vi "AndorTest.vi"() -> ()   [LabVIEW 2014]
uses:
  <userlib>/atmcd64d.llb/AcquisitionMode_mode typedef.ctl
  <userlib>/atmcd64d.llb/ReadMode_mode typedef.ctl
  <userlib>/atmcd64d.llb/Shutter_mode typedef.ctl
  <userlib>/atmcd64d.llb/Shutter_type typedef.ctl
  <userlib>/atmcd64d.llb/TriggerMode_mode typedef.ctl
  <userlib>/atmcd64d.llb/Error Code Enum typedef.ctl
panel:
  out "Waveform Chart":i32[][](graph)
  out "SetStatus":bool
  out "SetOut":T1
  out "Timing":T2 {"kinetic" format="%.2f"; "accumulate" format="%.2f"; "exposure" format="%.2f"}
  in  "MultiTrack":cluster{"StartRow":i32, "EndRow":i32}={"StartRow"=1, "EndRow"=256}
  in  "AcqSet":T3={"openingtime"=20, "closingtime"=20, "ExposureTime"=0.01, "AccumCycTime"=0.0, "AccumCycNum"=1, "KineticNum"=1, "KineticTime"=0.0} {"KineticTime" format="%.2f"; "AccumCycTime" format="%.2f"; "ExposureTime" format="%.2f"}
  in  "Mode":T9={"AcqMode"=enum."Single Scan", "ReadMode"=enum."Image", "ShutterMode"=enum."Auto", "GateMode"=enum."TTL High", "TriggerMode"=enum."Internal"}
  out "error out":errorcluster
  out "ShutDown":cluster{"CoolOff":bool, "ShutDown":bool}
  in  "stop":bool
  out "CoolerON":T10
  out "CurrentTemp":i32
  in  "TargetTemp":i32
  out "Speeds":T11
  out "SoftWVersion":T12
  out "HardWVersion":T13
  out "DevSize":cluster{"xpixels":i32, "ypixels":i32}
  out "DevInit":bool
  out "GetStatus":T14
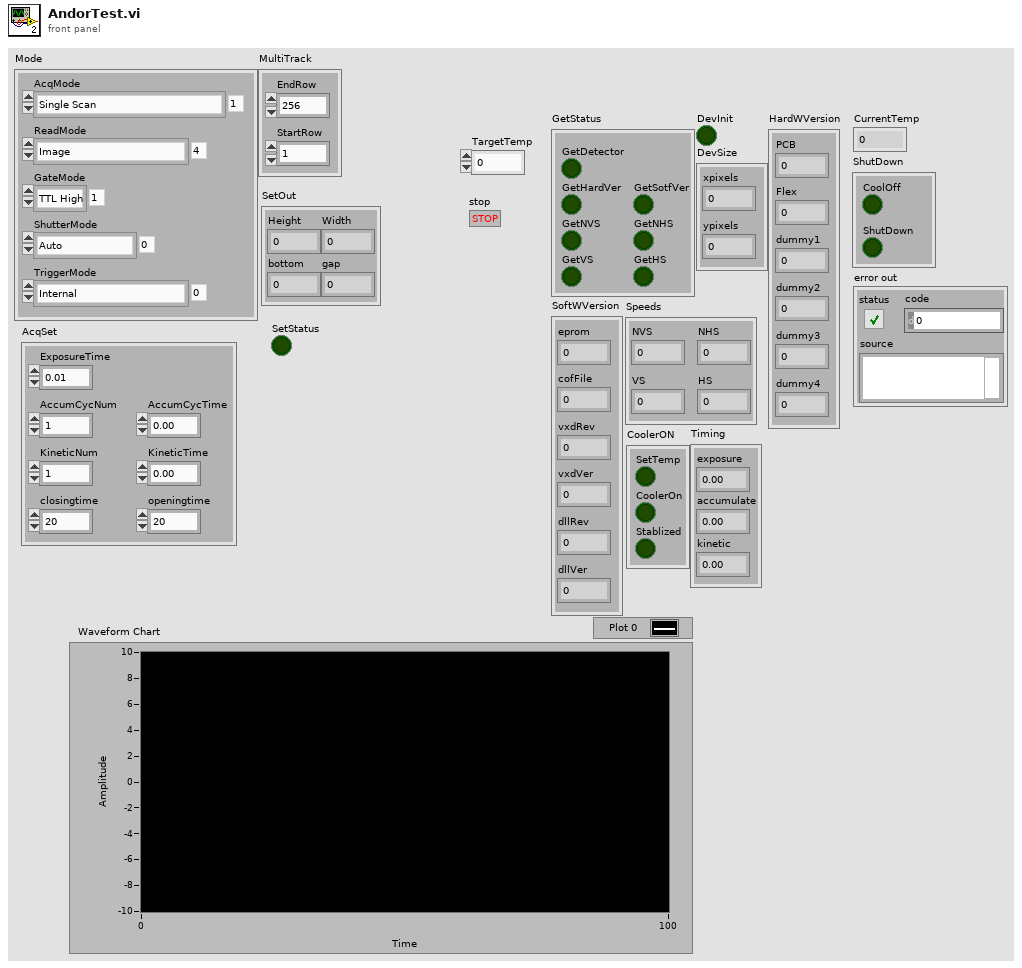
[diagram p1: front panel]
types:
  T1 = cluster{"Height":i32, "Width":i32, "bottom":i32, "gap":i32}
  T2 = cluster{"exposure":sgl, "accumulate":sgl, "kinetic":sgl}
  T3 = cluster{"openingtime":i32, "closingtime":i32, "ExposureTime":sgl, "AccumCycTime":sgl, "AccumCycNum":i32, "KineticNum":i32, "KineticTime":sgl}
  T4 = typedef "AcquisitionMode_mode typedef.ctl" = enum16{"Reserved (0)", "Single Scan", "Accumulate", "Kinetics", "Fast Kinetics", "Run Till Abort", "Reserved (6)", "Reserved (7)", "Reserved (8)", "Time Delayed Integration"}
  T5 = typedef "ReadMode_mode typedef.ctl" = enum16{"Full Vertical Binning", "Multi-Track", "Random-Track", "Single-Track", "Image"}
  T6 = typedef "Shutter_mode typedef.ctl" = enum16{"Auto", "Open", "Close", "N/A (3)", "Open FVB Series", "Open Any Series"}
  T7 = typedef "Shutter_type typedef.ctl" = enum16{"TTL Low", "TTL High"}
  T8 = typedef "TriggerMode_mode typedef.ctl" = enum16{"Internal", "External", "N/A (2)", "N/A (3)", "N/A (4)", "N/A (5)", "External Start", "External Exposure (Bulb)", "N/A (8)", "External FVB EM", "Software", "N/A (11)", "External Charge Shifting"}
  T9 = cluster{"AcqMode":T4, "ReadMode":T5, "ShutterMode":T6, "GateMode":T7, "TriggerMode":T8}
  T10 = cluster{"SetTemp":bool, "CoolerOn":bool, "Stablized":bool}
  T11 = cluster{"NVS":i32, "VS":i32, "NHS":dbl, "HS":i32}
  T12 = cluster{"eprom":u32, "cofFile":u32, "vxdRev":u32, "vxdVer":u32, "dllRev":u32, "dllVer":u32}
  T13 = cluster{"PCB":u32, "Flex":u32, "dummy1":u32, "dummy2":u32, "dummy3":u32, "dummy4":u32}
  T14 = cluster{"GetDetector":bool, "GetHardVer":bool, "GetNVS":bool, "GetVS":bool, "GetSotfVer":bool, "GetNHS":bool, "GetHS":bool}
  T15 = typedef "Error Code Enum typedef.ctl" = enum32{"N/A (0)", "DRV_ERROR_CODES", "DRV_SUCCESS", "DRV_VXDNOTINSTALLED", "DRV_ERROR_SCAN", "DRV_ERROR_CHECK_SUM", "DRV_ERROR_FILELOAD", "DRV_UNKNOWN_FUNC", "DRV_ERROR_VXD_INIT", "DRV_ERROR_ADDRESS", "DRV_ERROR_PAGELOCK", "DRV_ERROR_PAGEUNLOCK", "DRV_ERROR_BOARDTEST", "DRV_ERROR_ACK", "DRV_ERROR_UP_FIFO", "DRV_ERROR_PATTERN", "N/A (16)", "DRV_ACQUISITION_ERRORS", "DRV_ACQ_BUFFER", "DRV_ACQ_DOWNFIFO_FULL", "DRV_PROC_UNKONWN_INSTRUCTION", "DRV_ILLEGAL_OP_CODE", "DRV_KINETIC_TIME_NOT_MET", "DRV_ACCUM_TIME_NOT_MET", "DRV_NO_NEW_DATA", "N/A (25)", "DRV_SPOOLERROR", "N/A (27)", "N/A (28)", "N/A (29)", "N/A (30)", "N/A (31)", "N/A (32)", "DRV_TEMPERATURE_CODES", "DRV_TEMPERATURE_OFF", "DRV_TEMPERATURE_NOT_STABILIZED", "DRV_TEMPERATURE_STABILIZED", "DRV_TEMPERATURE_NOT_REACHED", "DRV_TEMPERATURE_OUT_RANGE", "DRV_TEMPERATURE_NOT_SUPPORTED", "DRV_TEMPERATURE_DRIFT", "N/A (41)", "N/A (42)", "N/A (43)", "N/A (44)", "N/A (45)", "N/A (46)", "N/A (47)", "N/A (48)", "DRV_GENERAL_ERRORS", "DRV_INVALID_AUX", "DRV_COF_NOTLOADED", "DRV_FPGAPROG", "DRV_FLEXERROR", "DRV_GPIBERROR", "N/A (55)", "N/A (56)", "N/A (57)", "N/A (58)", "N/A (59)", "N/A (60)", "N/A (61)", "N/A (62)", "N/A (63)", "DRV_DATATYPE", "DRV_DRIVER_ERRORS", "DRV_P1INVALID", "DRV_P2INVALID", "DRV_P3INVALID", "DRV_P4INVALID", "DRV_INIERROR", "DRV_COFERROR", "DRV_ACQUIRING", "DRV_IDLE", "DRV_TEMPCYCLE", "DRV_NOT_INITIALIZED", "DRV_P5INVALID", "DRV_P6INVALID", "DRV_INVALID_MODE", "DRV_INVALID_FILTER", "DRV_I2CERRORS", "DRV_I2CDEVNOTFOUND", "DRV_I2CTIMEOUT", "DRV_P7INVALID", "N/A (84)", "N/A (85)", "N/A (86)", "N/A (87)", "N/A (88)", "N/A (89)", "DRV_IOCERROR", "DRV_VRMVERSIONERROR"}
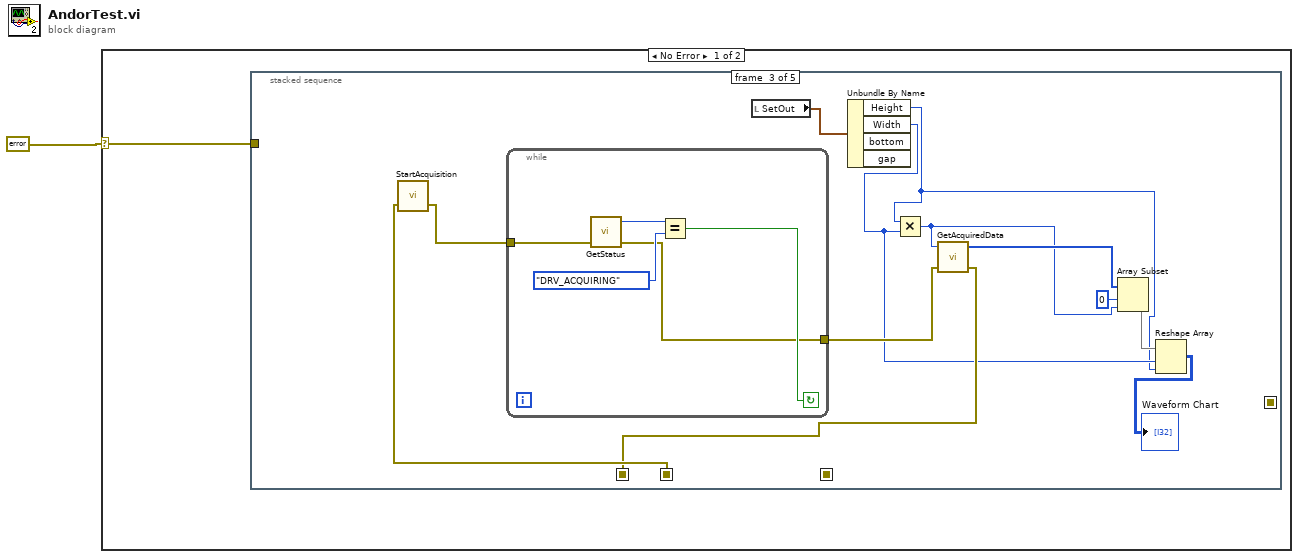
[diagram p0: block diagram]
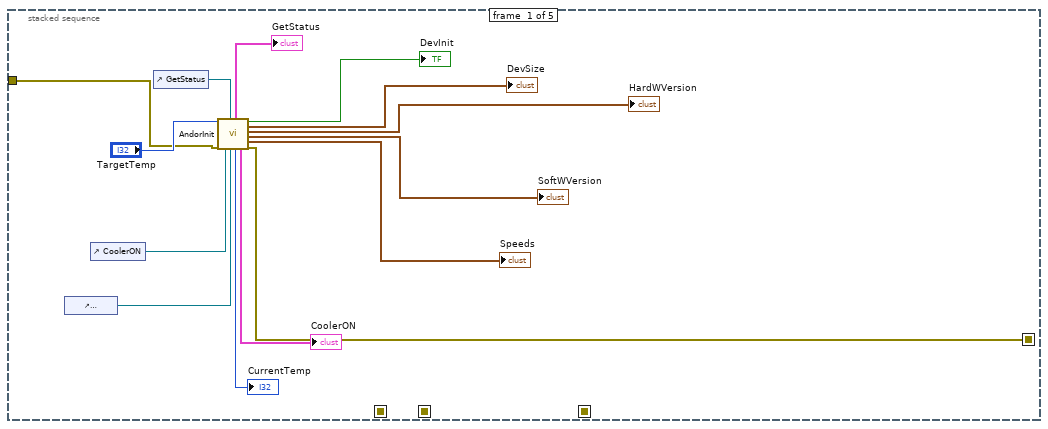
[diagram p2: hidden frame]
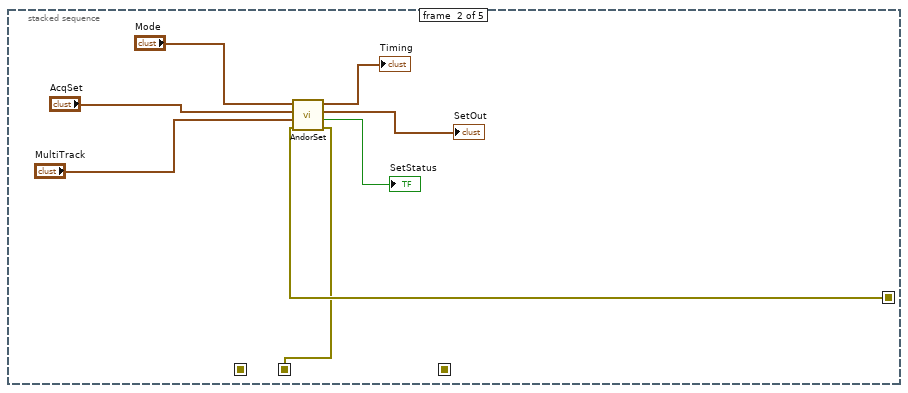
[diagram p3: hidden frame]
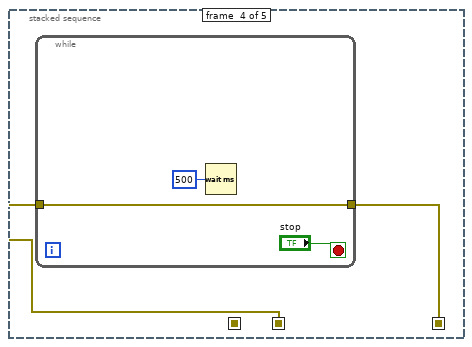
[diagram p4: hidden frame]
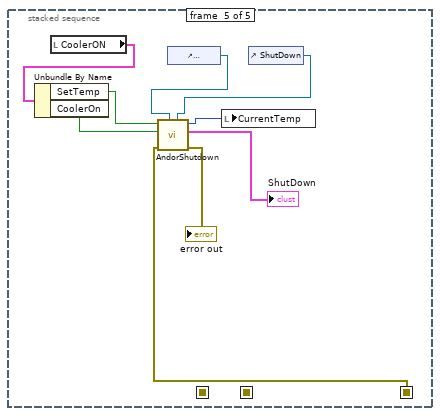
[diagram p5: hidden frame]
diagram:
  n1 = case shown="No Error" errorcluster {"status"=FALSE, "code"=0, "source"=""} ("error in (no error)") {
    selector: errorcluster {"status"=FALSE, "code"=0, "source"=""} ("error in (no error)") -> [w2 _]
    frame No Error {
      n2 = stacked-sequence {
        seq-local: [w4 _ _ _ _] -> [_ w21 _ _ _]
        seq-local: [_ w20 _ _ _] -> [_ _ w35 w43 _]
        seq-local: [_ _ w32 _ _] -> [_ _ _ _ _]
        seq-local: [_ _ _ w42 _] -> [_ _ _ _ w51]
        tunnel: w2 -> [w8 _ _ _ _]
        frame #0 {
          n3 = control-ref of="CurrentTemp"() -> (w5:refnum<vi>)
          n4 = control-ref of="CoolerON"() -> (w6:refnum<vi>)
          n5 = control-ref of="GetStatus"() -> (w15:refnum<vi>)
          n6 = call "AndorInit.vi"("TargetTemp"="TargetTemp", "error in"=w8, "CoolerONRef"=w6, "GetStatusRef"=w15, "CurrentTempRef"=w5) -> ("GetStatus"=→"GetStatus":T14, "CurrentTemp"=→"CurrentTemp":i32, "CoolerON"=→"CoolerON":T10, "DevInit"=→"DevInit":bool, "DevSize"=→"DevSize":cluster{"xpixels":i32, "ypixels":i32}, "HardWVersion"=→"HardWVersion":T13, "SoftWVersion"=→"SoftWVersion":T12, "Speeds"=→"Speeds":T11, "error out"=w4:errorcluster)  [unwired: 6 in]
        }
        frame #1 {
          n7 = call "AndorSet.vi"("error in"=w21, "MultiTrack"="MultiTrack", "AcqSet"="AcqSet", "Mode"="Mode") -> ("error out"=w20:errorcluster, "SetStatus"=→"SetStatus":bool, "SetOut"=→"SetOut":T1, "Timing"=→"Timing":T2)  [unwired: 4 in]
        }
        frame #2 {
          n8 = call <userlib>:"StartAcquisition.vi"("error in (no error)"=w35) -> ("error out"=w36:errorcluster)  [unwired: 1 in, 1 out]
          n9 = while {
            tunnel: w36 -> [w41]
            tunnel: [w37] -> w34
            stop <- w38 continue-if-true
            n10 = call <userlib>:"GetStatus.vi"("error in (no error)"=w41) -> ("error out"=w37:errorcluster, "status"=w40:T15)  [unwired: 2 in, 1 out]
            n11 = Equal?(x=w40, y=Error_Code_Enum_typedef."DRV_ACQUIRING") -> (x = y?=w38:bool)
          }
          n12 = local read "SetOut"() -> (w33:T1)
          n13 = Unbundle By Name(w33) -> ("Height"=w26:i32, "Width"=w27:i32)  [unwired: 2 out]
          n14 = Multiply(x=w26, y=w27) -> (x*y=w29:i32)
          n15 = call <userlib>:"GetAcquiredData.vi"("error in (no error)"=w34, "size"=w29) -> ("error out"=w32:errorcluster, "array"=w31:i32[])  [unwired: 1 in, 1 out]
          n16 = Array Subset(array=w31, index=0, length=w29) -> (w28:i32[])
          n17 = Reshape Array(w28, w27, w26) -> (→"Waveform Chart":i32[][])
        }
        frame #3 {
          n18 = while {
            tunnel: [w44] -> w42
            tunnel: w43 -> [w44]
            stop <- "stop" stop-if-true
            n19 = Wait (ms)(milliseconds to wait=u32 500) -> ()  [unwired: 1 out]
          }
        }
        frame #4 {
          n20 = local read "CoolerON"() -> (w50:T10)
          n21 = Unbundle By Name(w50) -> ("SetTemp"=w49:bool, "CoolerOn"=w48:bool)
          n22 = control-ref of="CurrentTemp"() -> (w55:refnum<vi>)
          n23 = control-ref of="ShutDown"() -> (w47:refnum<vi>)
          n24 = call "AndorShutdown.vi"("ShutDownRef"=w47, "CurrentTempRef"=w55, "error in"=w51, "CoolerON"=w48, "SetTemp"=w49) -> ("error out"=→"error out":errorcluster, "ShutDown"=→"ShutDown":cluster{"CoolOff":bool, "ShutDown":bool}, "CurrentTemp"=w54:i32)  [unwired: 4 in]
          n25 = local write "CurrentTemp"(w54) -> ()
        }
      }
    }
    frame Error {
    }
  }
